vi "Receive Batch Node Actors VI Ref.vi"(6 "Paras In":variant, 7 "Actors In":refnum<class "System Actor.lvclass">[](array[class]), 8 "error in (no error)":errorcluster, 10 "VI Refs In":refnum<vi>[](array[refnum]), 11 "Node Controller in":refnum<class "Node Controller.lvclass">) -> (0 "error out":errorcluster, 3 "Node Controller out":refnum<class "Node Controller.lvclass">, 5 "Actors Out":refnum<class "System Actor.lvclass">[](array[class]))   [LabVIEW 2024, in "Node Controller.lvclass"]
uses:
  Node Controller.lvclass
  Messenger/Mail Strategy/Mail Strategy.lvclass
  Actor/System Actor/System Actor.lvclass
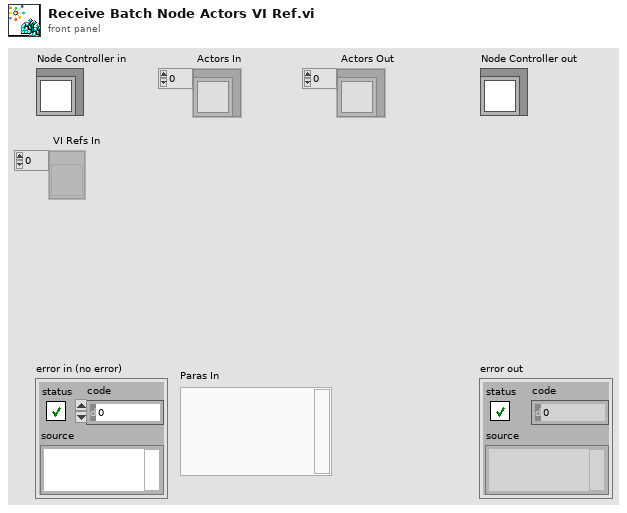
[diagram p1: front panel]
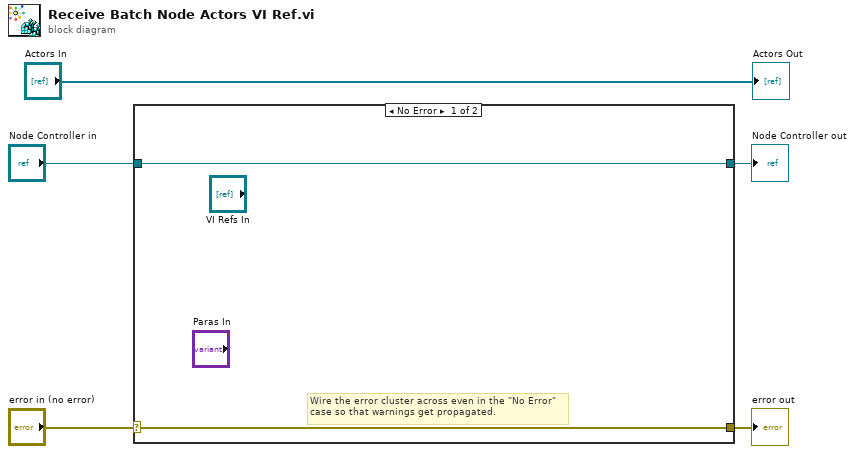
[diagram p0: block diagram]
diagram:
  n1 = case shown="No Error" "error in (no error)" {
    selector: "error in (no error)" -> [w6 w9]
    tunnel: [w6 w9] -> w4
    tunnel: [w7 w8] -> w2
    tunnel: "Node Controller in" -> [w7 w8]
    frame No Error {
      # "Wire the error cluster across even in the \"No Error\"\ncase so that warnings get propagated."
    }
    frame Error {
    }
  }
  "error out" <- w4
  "Node Controller out" <- w2
  "Actors Out" <- "Actors In"
